vi "enum_to_error_code.vi"(4 "Error Enum in":T1=enum."VISA_err_Timeout") -> (1 "error code out":i32)   [LabVIEW 2022 SP3, in "hmp4000_rsidr_core.lvlib"]
uses:
  hmp4000_rsidr_core.lvlib
  type_Error_Codes.ctl
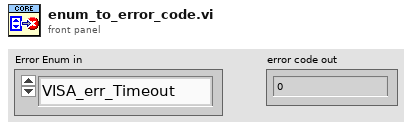
[diagram p1: front panel]
types:
  T1 = typedef "hmp4000_rsidr_core.lvlib/type_Error_Codes.ctl" = enum16{"No_error", "VISA_err_ResourceNotFound", "VISA_err_Timeout", "VISA_warn_MoreDataAvailable", "RS_err_MissingCallback", "RS_err_InvalidAttribute", "RS_err_InvalidValue", "RS_err_UnknownResource", "RS_err_AlreadyInitialized", "RS_err_InstrumentStatus", "RS_err_BadRepCapName", "RS_err_TypesMismatch", "RS_err_ValueNotSupported", "RS_err_InvalidRngTable", "RS_err_IDqueryFail", "RS_err_UnexpResponse", "VISA_warn_ConfigNotLoaded", "RS_err_AttributeNotReadable", "RS_err_AttributeNotWritable", "RS_err_InstrumentType", "RS_err_InstrumentOption", "VISA_err_InvalidSize", "RS_err_ReliabilityIndicator", "VISA_warn_UnknownStatus", "VISA_warn_TermCharRead", "VISA_err_IO_error", "RS_err_FunctionNotSupported", "VISA_warn_QueueEmpty"}
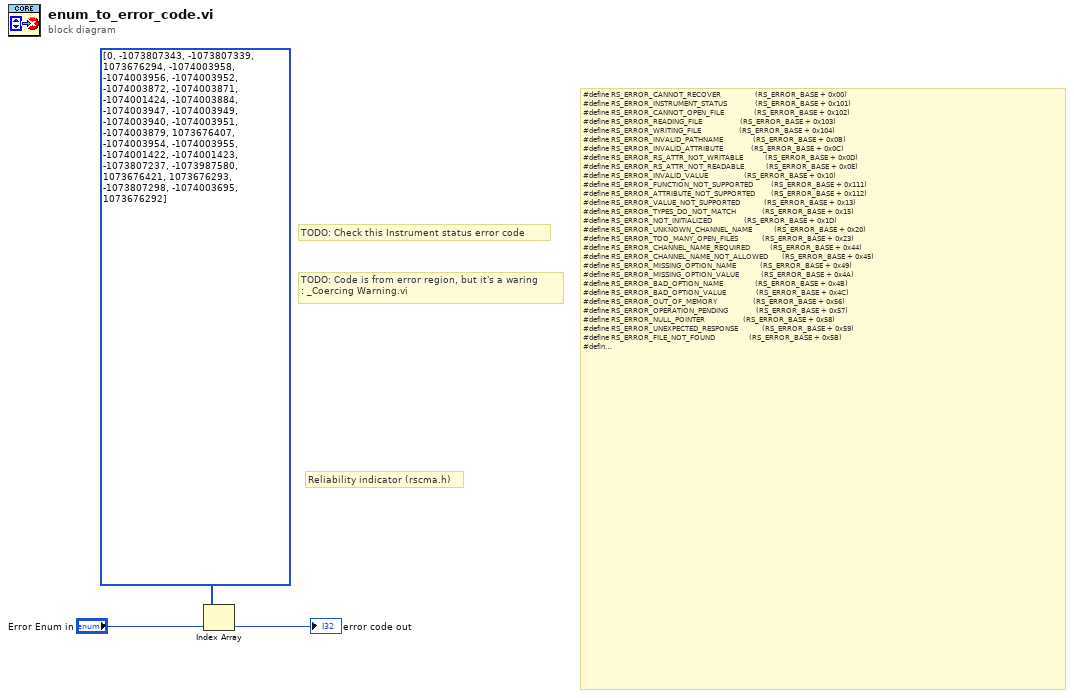
[diagram p0: block diagram]
diagram:
  # "TODO: Code is from error region, but it's a waring\n: _Coercing Warning.vi"
  # "Reliability indicator (rscma.h)"
  # "TODO: Check this Instrument status error code"
  # "#define RS_ERROR_CANNOT_RECOVER                 (RS_ERROR_BASE + 0x00)\n#define RS_ERROR_INSTRUMENT_STATUS              (RS_ERROR_BASE + 0x101)\n#define RS_ERROR_CANNOT_OPEN_FILE               (RS_ERROR_BASE + 0x102)\n#define RS_ERROR_READING_FILE                   (RS_ERROR_BASE + 0x103)\n#define RS_ERROR_WRITING_FILE                   (RS_ERROR_BASE + 0x104)\n#define RS_ERROR_INVALID_PATHNAME               (RS_ERROR_BASE + 0x0B)\n#define RS_ERROR_INVALID_ATTRIBUTE              (RS_ERROR_BASE + 0x0C)\n#define RS_ERROR_RS_ATTR_NOT_WRITABLE           (RS_ERROR_BASE + 0x0D)\n#define RS_ERROR_RS_ATTR_NOT_READABLE           (RS_ERROR_BASE + 0x0E)\n#define RS_ERROR_INVALID_VALUE                  (RS_ERROR_BASE + 0x10)\n#define RS_ERROR_FUNCTION_NOT_SUPPORTED         (RS_ERROR_BASE + 0x111)\n#define RS_ERROR_ATTRIBUTE_NOT_SUPPORTED        (RS_ERROR_BASE + 0x112)\n#define RS_ERROR_VALUE_NOT_SUPPORTED            (RS_ERROR_BASE + 0x13)\n#define RS_ERROR_TYPES_DO_NOT_MATCH             (RS_ERROR_BASE + 0x15)\n#define RS_ERROR_NOT_INITIALIZED                (RS_ERROR_BASE + 0x1D)\n#define RS_ERROR_UNKNOWN_CHANNEL_NAME           (RS_ERROR_BASE + 0x20)\n#define RS_ERROR_TOO_MANY_OPEN_FILES            (RS_ERROR_BASE + 0x23)\n#define RS_ERROR_CHANNEL_NAME_REQUIRED          (RS_ERROR_BASE + 0x44)\n#define RS_ERROR_CHANNEL_NAME_NOT_ALLOWED       (RS_ERROR_BASE + 0x45)\n#define RS_ERROR_MISSING_OPTION_NAME            (RS_ERROR_BASE + 0x49)\n#define RS_ERROR_MISSING_OPTION_VALUE           (RS_ERROR_BASE + 0x4A)\n#define RS_ERROR_BAD_OPTION_NAME                (RS_ERROR_BASE + 0x4B)\n#define RS_ERROR_BAD_OPTION_VALUE               (RS_ERROR_BASE + 0x4C)\n#define RS_ERROR_OUT_OF_MEMORY                  (RS_ERROR_BASE + 0x56)\n#define RS_ERROR_OPERATION_PENDING              (RS_ERROR_BASE + 0x57)\n#define RS_ERROR_NULL_POINTER                   (RS_ERROR_BASE + 0x58)\n#define RS_ERROR_UNEXPECTED_RESPONSE            (RS_ERROR_BASE + 0x59)\n#define RS_ERROR_FILE_NOT_FOUND                 (RS_ERROR_BASE + 0x5B)\n#define RS_ERROR_INVALID_FILE_FORMAT            (RS_ERROR_BASE + 0x5C)\n#define RS_ERROR_STATUS_NOT_AVAILABLE           (RS_ERROR_BASE + 0x5D)\n#define RS_ERROR_ID_QUERY_FAILED                (RS_ERROR_BASE + 0x5E)\n#define RS_ERROR_RESET_FAILED                   (RS_ERROR_BASE + 0x5F)\n#define RS_ERROR_RESOURCE_UNKNOWN               (RS_ERROR_BASE + 0x60)\n#define RS_ERROR_ALREADY_INITIALIZED            (RS_ERROR_BASE + 0x61)\n#define RS_ERROR_CANNOT_CHANGE_SIMULATION_STATE         (RS_ERROR_BASE + 0x62)\n#define RS_ERROR_INVALID_NUMBER_OF_LEVELS_IN_SELECTOR   (RS_ERROR_BASE + 0x63)\n#define RS_ERROR_INVALID_RANGE_IN_SELECTOR      (RS_ERROR_BASE + 0x64)\n#define RS_ERROR_UNKOWN_NAME_IN_SELECTOR        (RS_ERROR_BASE + 0x65)\n#define RS_ERROR_BADLY_FORMED_SELECTOR          (RS_ERROR_BASE + 0x66)\n#define RS_ERROR_UNKNOWN_PHYSICAL_IDENTIFIER    (RS_ERROR_BASE + 0x67)"
  n1 = Index Array(array=i32[] [0, -1073807343, -1073807339, 1073676294, -1074003958, -1074003956, -1074003952, -1074003872, -1074003871, -1074001424, -1074003884, -1074003947, -1074003949, -1074003940, -1074003951, -1074003879, 1073676407, -1074003954, -1074003955, -1074001422, -1074001423, -1073807237, -1073987580, 1073676421, 1073676293, -1073807298, -1074003695, 1073676292], index="Error Enum in") -> (element=→"error code out":i32)
